vi "Pulse_Memory_buton.vi"(3 "Reset":bool, 6 "Pulse":bool) -> (1 "Memory":bool)   [LabVIEW 2017]
doc: "Recibe un pulso boleano (Pulse) y cambia de estado una salida boleana (Memory). Necesita del aestado anerior"
panel:
  out "MemoIn":bool
  out "Pulse_delay":bool
  out "Valor anterioro":bool
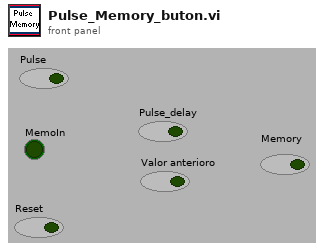
[diagram p1: front panel]
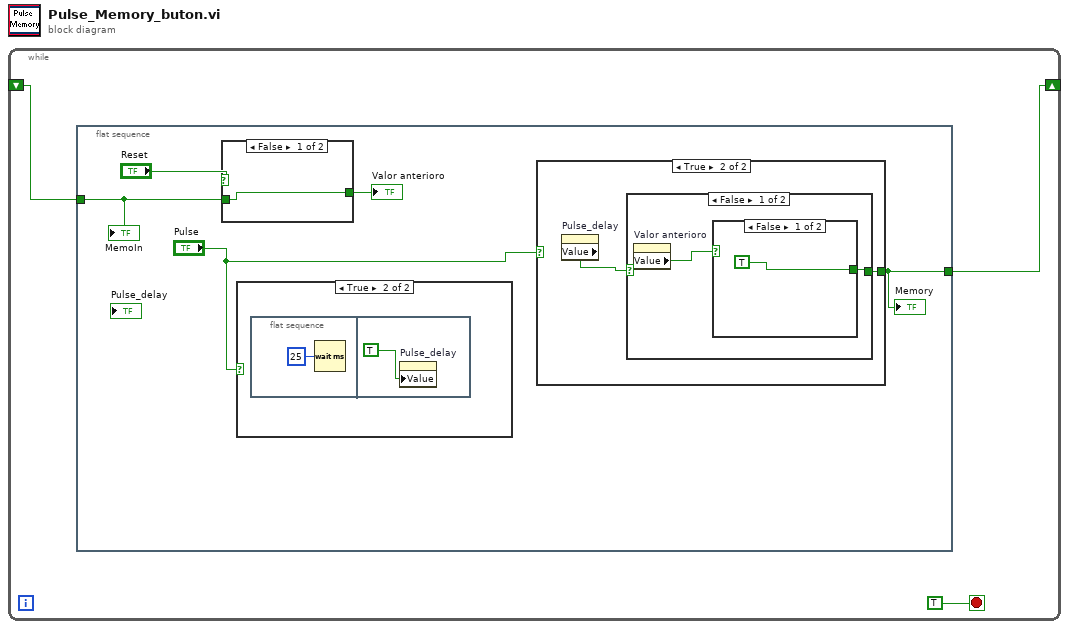
[diagram p0: block diagram]
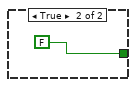
[diagram p2: hidden frame]
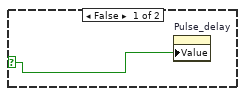
[diagram p3: hidden frame]
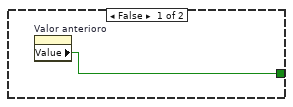
[diagram p4: hidden frame]
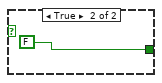
[diagram p5: hidden frame]
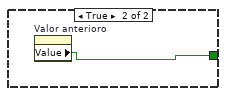
[diagram p6: hidden frame]
diagram:
  n1 = while {
    shift-right: [w1] -> _
    shift-left: _ -> [w2]
    stop <- TRUE stop-if-true
    n2 = flat-sequence {
      tunnel: [w4] -> w1
      tunnel: w2 -> [w6]
      frame #0 {
        n3 = case shown="False" "Reset" {
          tunnel: w6 -> [w9 _]
          tunnel: [w9 FALSE] -> w5
          frame False {
          }
          frame True {
          }
        }
        "Valor anterioro" <- w5
        n4 = case shown="True" "Pulse" {
          selector: "Pulse" -> [w11 _]
          frame False {
            n5 = property on="Pulse_delay" class="Bool (strict)"("Value"=w11) -> ()  [unwired: 2 in, 2 out]
          }
          frame True {
            n6 = flat-sequence {
              frame #0 {
                n7 = Wait (ms)(milliseconds to wait=u32 25) -> ()  [unwired: 1 out]
              }
              frame #1 {
                n8 = property on="Pulse_delay" class="Bool (strict)"("Value"=TRUE) -> ()  [unwired: 2 in, 2 out]
              }
            }
          }
        }
        n9 = case shown="True" "Pulse" {
          tunnel: [w14 w15] -> w4
          frame False {
            n10 = property on="Valor anterioro" class="Bool (strict)"() -> ("Value"=w14:bool)  [unwired: 2 in, 2 out]
          }
          frame True {
            n11 = property on="Pulse_delay" class="Bool (strict)"() -> ("Value"=w16:bool)  [unwired: 2 in, 2 out]
            n12 = case shown="False" w16 {
              tunnel: [w17 w21] -> w15
              frame False {
                n13 = property on="Valor anterioro" class="Bool (strict)"() -> ("Value"=w18:bool)  [unwired: 2 in, 2 out]
                n14 = case shown="False" w18 {
                  tunnel: [TRUE FALSE] -> w17
                  frame False {
                  }
                  frame True {
                  }
                }
              }
              frame True {
                n15 = property on="Valor anterioro" class="Bool (strict)"() -> ("Value"=w21:bool)  [unwired: 2 in, 2 out]
              }
            }
          }
        }
        "Memory" <- w4
        "MemoIn" <- w6
      }
    }
  }
